vi "2FT.vi"(7 "error in":errorcluster) -> (20 "Matches (Geometric Matching 1)":T2[](array[typedef]) {"Correlation Score" format="%.2f"; "Target Template Curve Score" format="%.2f"; "Template Target Curve Score" format="%.2f"; "Bounding Box"."y" format="%.2f"; "Bounding Box"."x" format="%.2f"; "Position"."y" format="%.2f"; "Position"."x" format="%.2f"; "Score" format="%.2f"; "Scale" format="%.2f"; "Angle" format="%.2f"; "Occlusion %" format="%.2f"}, 21 "Calibrated Matches (Geometric Matching 1)":T2[](array[typedef]) {"Correlation Score" format="%.2f"; "Target Template Curve Score" format="%.2f"; "Template Target Curve Score" format="%.2f"; "Bounding Box"."y" format="%.2f"; "Bounding Box"."x" format="%.2f"; "Position"."y" format="%.2f"; "Position"."x" format="%.2f"; "Score" format="%.2f"; "Scale" format="%.2f"; "Angle" format="%.2f"; "Occlusion %" format="%.2f"}, 22 "Number of Matches (Geometric Matching 1)":i32, 27 "error out":errorcluster)   [LabVIEW 2016]
uses:
  <vilib>/vision/Pattern Matching.llb/IMAQ GM Match Report.ctl
  <vilib>/vision/Image Controls.llb/Vision Info Type2.ctl
  <vilib>/vision/Pattern Matching.llb/IMAQ Curve Parameters.ctl
  <vilib>/vision/Pattern Matching.llb/IMAQ Match Range Setting.ctl
  <vilib>/vision/driver/NI_Vision_Acquisition_Software.lvlib
  <vilib>/vision/NI_Vision_Development_Module.lvlib
panel:
  out "Image Out":T1(plugin-control)
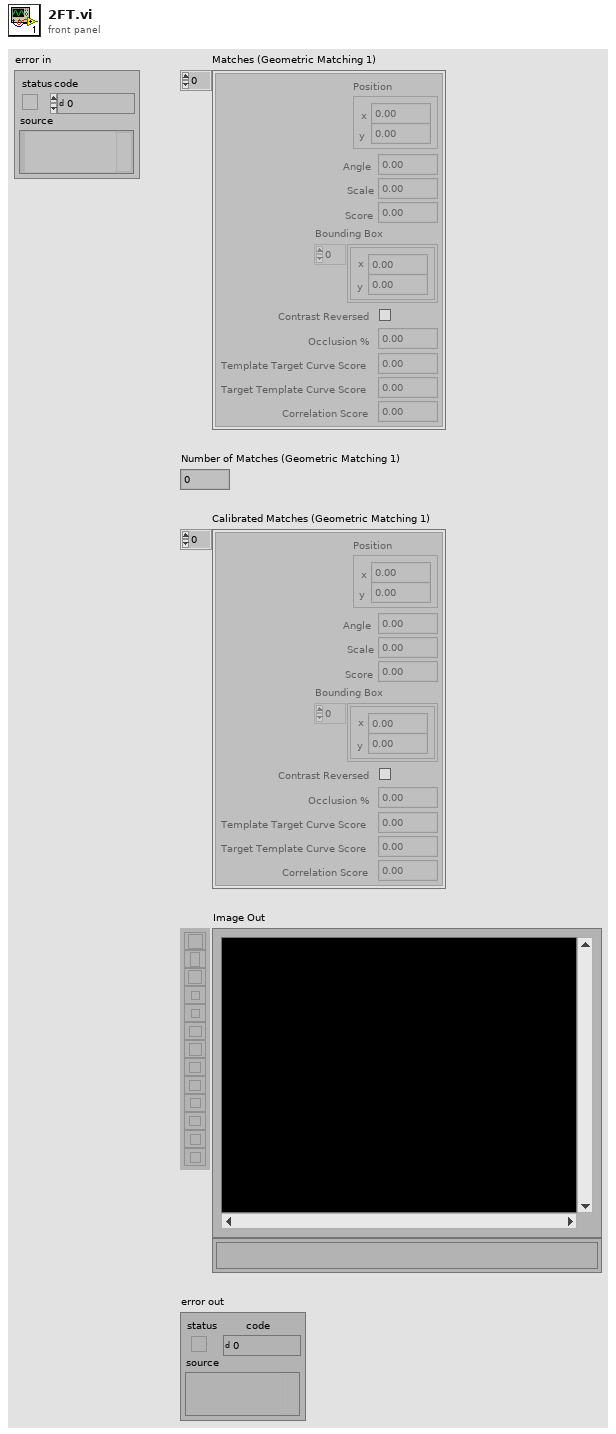
[diagram p1: front panel]
types:
  T1 = typedef "IMAQ Image.ctl" = refnum<image>
  T2 = typedef "IMAQ GM Match Report.ctl" = cluster{"Position":cluster{"x":sgl, "y":sgl}, "Angle":sgl, "Scale":sgl, "Score":sgl, "Bounding Box":cluster{"x":sgl, "y":sgl}[], "Contrast Reversed":bool, "Occlusion %":sgl, "Template Target Curve Score":sgl, "Target Template Curve Score":sgl, "Correlation Score":sgl}
  T3 = typedef "IMAQ Curve Parameters.ctl" = cluster{"Extraction Mode":u32, "Edge Threshold":i32, "Edge Filter Size":u32, "Min Length":i32, "Row Search Step Size":i32, "Col Search Step Size":i32, "Max Endpoint Gap":i32, "Closed":bool, "Subpixel":bool}
  T4 = typedef "IMAQ Match Range Setting.ctl" = cluster{"Match Constraints":u32, "Min":dbl, "Max":dbl}
  T5 = cluster{"Curve Parameters":T3, "Match Mode":cluster{"Rotation":bool, "Scale":bool, "Occlusion":bool, "Reserved":bool, "Reserved":bool, "Reserved":bool}, "Range Settings":T4[], "Number of Matches":i32, "Minimum Match Score":sgl, "SubPixel Accuracy":bool, "Adv. Geometric Match Options 2":cluster{"Setup Data Item":u16, "Item Value":dbl}[]}
  T6 = cluster{"Global Rectangle":i32[], "Contours":cluster{"ID":enum32{"External", "Internal"}, "Type":u32, "Coordinates":i32[]}[]}
  T7 = typedef "Vision Info Type2.ctl" = u32
  T8 = cluster{"Origin Pixel":cluster{"X":sgl, "Y":sgl}, "Angle Relative to Horizontal (deg)":sgl, "Axis Reference":u32}
  T9 = enum32{"AutoM", "Close", "Dilate", "Erode", "Gradient", "Gradient out", "Gradient in", "Hit miss", "Open", "PClose", "POpen", "Thick", "Thin"}
  T10 = cluster{"Brightness":sgl, "Contrast":sgl, "Gamma":sgl}
  T11 = typedef "IMAQdx.ctl" = refnum<k21>
  T12 = cluster{"histogram":u32[], "Minimal Value":sgl, "Maximal Value":sgl, "Starting Value":sgl, "Interval Width":sgl, "Mean Value":sgl, "Standard  Variation":sgl, "Area (pixels)":i32}
  T13 = typedef "Image Type" = u32
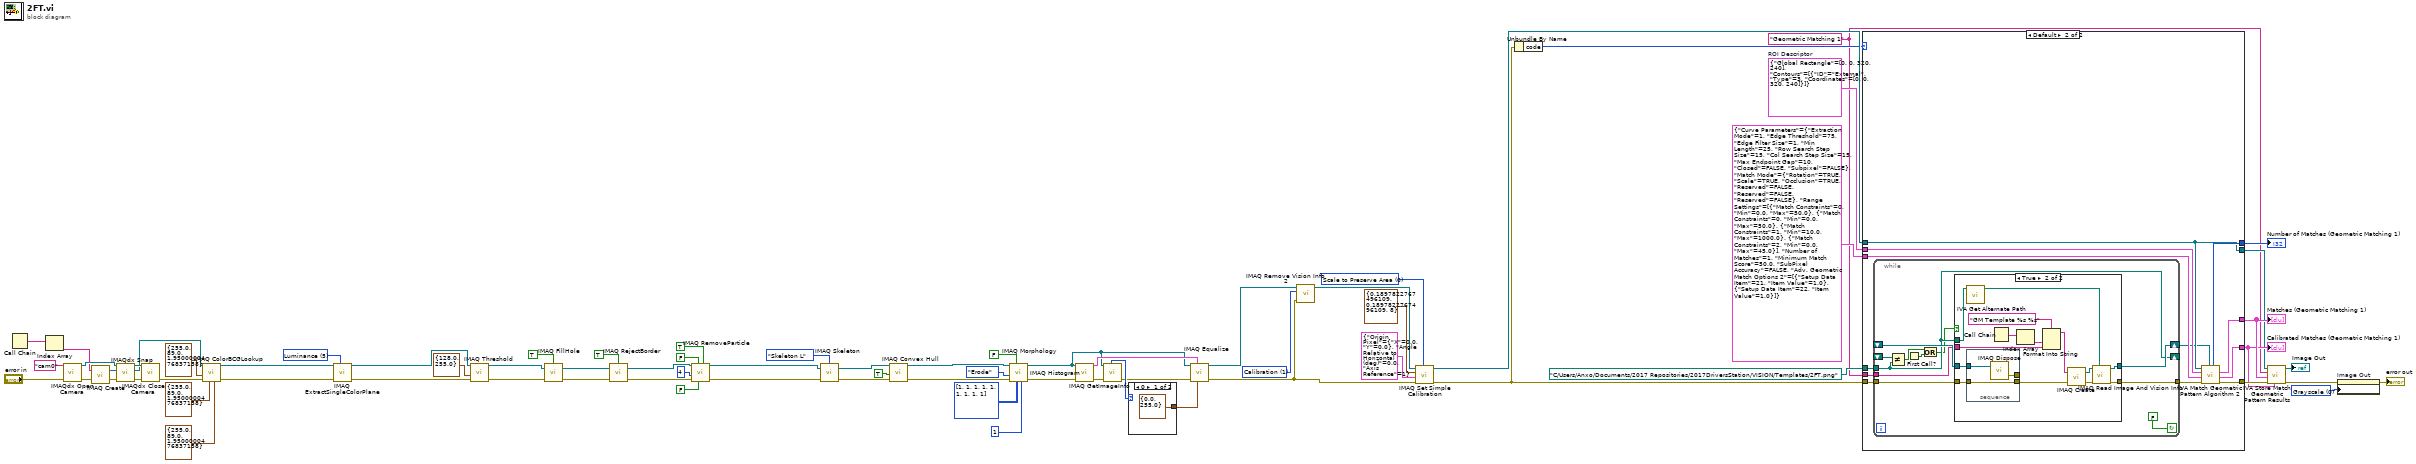
[diagram p0: block diagram]
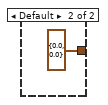
[diagram p4: hidden frame]
diagram:
  w1 = u32 0 items=["Grayscale", "Binary", "Gradient", "Rainbow", "Temperature", "User Defined", "Binary 16 Bit", "Gradient 16 Bit", "Rainbow 16 Bit", "Temperature 16 Bit", "User Defined 16 Bit"] ("Palette Type")
  w5 = "Geometric Matching 1" ("Step Name")
  w15 = T6 {"Global Rectangle"=[0, 0, 320, 240], "Contours"=[{"ID"=enum."External", "Type"=3, "Coordinates"=[0, 0, 320, 240]}]}  # ROI Descriptor
  w18 = T7 1 items=["Any", "Calibration", "Overlay", "Grayscale Template", "Color Template", "Geometric Template", "Custom Data", "Golden Template", "Geometric Template 2", "Contour Data", "Camera Model"] ("Vision Info")
  w23 = u32 0 items=["Scale to Preserve Area", "Scale to Fit"] ("Corrected Image Scaling")
  w60 = 5 items=["Red", "Green", "Blue", "Hue", "Saturation", "Luminance", "Value", "Intensity"] ("Color Plane")
  n1 = Call Chain() -> (call chain=w67:string[])
  n2 = Index Array(array=w67) -> (element=w66:string)  [unwired: 1 in]
  n3 = call <vilib>:"IMAQdx Open Camera.vi"("error in"="error in", "Session In"="cam0" ("Interface Name")) -> ("error out"=w74:errorcluster, "Session Out"=w69:T11)  [unwired: 1 in, 7 out]
  n4 = call "IMAQ Create"("Image Name"=w66, "error in (no error)"=w74) -> ("New Image"=w71:T1, "error out"=w70:errorcluster)  [unwired: 2 in, 1 out]
  n5 = call <vilib>:"IMAQdx Snap.vi"("error in"=w70, "Image In"=w71, "Session In"=w69) -> ("error out"=w72:errorcluster, "Image Out"=w65:T1, "Session Out"=w73:T11)  [unwired: 6 out]
  n6 = call <vilib>:"IMAQdx Close Camera.vi"("error in"=w72, "Session In"=w73) -> ("error out"=w64:errorcluster)  [unwired: 9 out]
  n7 = call "IMAQ ColorBCGLookup"("Blue BCG Values"=T10 {"Brightness"=255.0, "Contrast"=89.0, "Gamma"=1.95}, "Green BCG Values"=T10 {"Brightness"=255.0, "Contrast"=89.0, "Gamma"=1.95}, "error in (no error)"=w64, "Red BCG Values"=T10 {"Brightness"=255.0, "Contrast"=89.0, "Gamma"=1.95}, "Image Src"=w65) -> ("error out"=w58:errorcluster, "Image Dst Out"=w59:T1)  [unwired: 2 in, 3 out]
  n8 = call "IMAQ ExtractSingleColorPlane"("Color Plane"=w60, "error in (no error)"=w58, "Image Src"=w59) -> ("error out"=w55:errorcluster, "Image Dst Out"=w56:T1)  [unwired: 1 in, 6 out]
  n9 = call "IMAQ Threshold"("error in (no error)"=w55, "Range"=cluster{"Lower value":sgl, "Upper value":sgl} {"Lower value"=128.0, "Upper value"=255.0}, "Image Src"=w56) -> ("error out"=w52:errorcluster, "Image Dst Out"=w53:T1)  [unwired: 3 in, 4 out]
  n10 = call "IMAQ FillHole"("error in (no error)"=w52, "Image Src"=w53, "Connectivity 4/8 (8)"=TRUE) -> ("error out"=w49:errorcluster, "Image Dst Out"=w50:T1)  [unwired: 1 in, 2 out]
  n11 = call "IMAQ RejectBorder"("error in (no error)"=w49, "Image Src"=w50, "Connectivity 4/8 (8)"=TRUE) -> ("error out"=w43:errorcluster, "Image Dst Out"=w44:T1)  [unwired: 1 in, 2 out]
  n12 = call "IMAQ RemoveParticle"("Connectivity 4/8 (8)"=TRUE, "Low Pass/High Pass (Low)"=FALSE, "Square/Hexa (Square)"=FALSE, "error in (no error)"=w43, "Number of Erosion"=4, "Image Src"=w44) -> ("error out"=w40:errorcluster, "Image Dst Out"=w41:T1)  [unwired: 1 in, 3 out]
  n13 = call "IMAQ Skeleton"("error in (no error)"=w40, "Image Src"=w41, "Mode"=enum32{"Skeleton L", "Skeleton M", "Skiz"}."Skeleton L") -> ("error out"=w38:errorcluster, "Image Dst Out"=w39:T1)  [unwired: 1 in, 2 out]
  n14 = call "IMAQ Convex Hull"("error in (no error)"=w38, "Connectivity 4/8 (8)"=TRUE, "Image Src"=w39) -> ("error out"=w31:errorcluster, "Image Dst Out"=w32:T1)  [unwired: 1 in, 6 out]
  n15 = call "IMAQ Morphology"("Number of iterations (1)"=1, "Structuring Element"=i32[][] [[1, 1, 1], [1, 1, 1], [1, 1, 1]], "Square/Hexa (Square)"=FALSE, "error in (no error)"=w31, "Operation"=T9."Erode", "Image Src"=w32) -> ("error out"=w29:errorcluster, "Image Dst Out"=w27:T1)  [unwired: 1 in, 3 out]
  n16 = call "IMAQ Histogram"("error in (no error)"=w29, "Image"=w27) -> ("error out"=w26:errorcluster, "Histogram Report"=w30:T12)  [unwired: 3 in, 5 out]
  n17 = call "IMAQ GetImageInfo"("error in (no error)"=w26, "Image"=w27) -> ("error out"=w25:errorcluster, "Image Type"=w28:T13)  [unwired: 8 out]
  n18 = case shown="0" w28 {
    tunnel: [cluster{"Minimum":sgl, "Maximum":sgl} {"Minimum"=0.0, "Maximum"=255.0} ("Range") cluster{"Minimum":sgl, "Maximum":sgl} {"Minimum"=0.0, "Maximum"=0.0} ("Range")] -> w24
    frame 0 {
    }
    frame Default {
    }
  }
  n19 = call "IMAQ Equalize"("Range"=w24, "Histogram Report"=w30, "error in (no error)"=w25, "Image Src"=w27) -> ("error out"=w17:errorcluster, "Image Dst Out"=w20:T1)  [unwired: 2 in, 4 out]
  n20 = call "IMAQ Remove Vision Info 2"("error in (no error)"=w17, "Vision Info"=w18, "Image"=w20) -> ("Image Out"=w19:T1)  [unwired: 8 out]
  n21 = call "IMAQ Set Simple Calibration"("Corrected Image Scaling"=w23, "error in (no error)"=w17, "Calibration Axis Info"=T8 {"Origin Pixel"={"X"=0.0, "Y"=0.0}, "Angle Relative to Horizontal (deg)"=0.0, "Axis Reference"=1}, "Grid Descriptor"=cluster{"X Step":sgl, "Y Step":sgl, "Unit":u32} {"X Step"=0.18978228, "Y Step"=0.18978228, "Unit"=8}, "Image"=w19) -> ("error out"=w9:errorcluster, "Calibrated Image"=w14:T1)  [unwired: 1 in, 4 out]
  n22 = Unbundle By Name(w9) -> ("code"=w8:i32)
  n23 = case shown="Default" w8 {
    tunnel: path "C:/Users/Anxo/Documents/2017 Repositories/2017DriversStation/VISION/Templates/2FT.png" ("Template File Path") -> [_ w83]
    tunnel: w9 -> [_ w82]
    tunnel: T5 {"Curve Parameters"={"Extraction Mode"=1, "Edge Threshold"=75, "Edge Filter Size"=1, "Min Length"=25, "Row Search Step Size"=15, "Col Search Step Size"=15, "Max Endpoint Gap"=10, "Closed"=FALSE, "Subpixel"=FALSE}, "Match Mode"={"Rotation"=TRUE, "Scale"=TRUE, "Occlusion"=TRUE, "Reserved"=FALSE, "Reserved"=FALSE, "Reserved"=FALSE}, "Range Settings"=[{"Match Constraints"=0, "Min"=0.0, "Max"=50.0}, {"Match Constraints"=0, "Min"=0.0, "Max"=50.0}, {"Match Constraints"=1, "Min"=10.0, "Max"=1000.0}, {"Match Constraints"=2, "Min"=0.0, "Max"=45.0}], "Number of Matches"=1, "Minimum Match Score"=50.0, "SubPixel Accuracy"=FALSE, "Adv. Geometric Match Options 2"=[{"Setup Data Item"=21, "Item Value"=1.0}, {"Setup Data Item"=22, "Item Value"=1.0}]} ("Settings") -> [_ w90]
    tunnel: w15 -> [_ w89]
    tunnel: w14 -> [w78 w84]
    tunnel: [_ w88] -> w13
    tunnel: [_ w87] -> w12
    tunnel: [_ w86] -> w11
    tunnel: [_ w85] -> w10
    tunnel: [w78 w84] -> w7
    tunnel: w5 -> [_ w79]
    frame -1074396199, -1074396198 {
      # "Discard Coordinate System Error"
    }
    frame Default {
      n24 = while {
        shift-right: [w101] -> w80
        shift-left: _ -> [w100]
        tunnel: [w98] -> w81
        tunnel: w82 -> [w97]
        tunnel: w83 -> [w94]
        tunnel: w79 -> [w96]
        shift-right: [w94] -> _
        shift-left: _ -> [w95]
        stop <- FALSE continue-if-true
        n25 = Not Equal?(x=w95, y=w94) -> (x != y?=w92:bool)
        n26 = First Call?() -> (First Call?: T/F=w93:bool)
        n27 = Or(x=w92, y=w93) -> (x .or. y?=w91:bool)
        n28 = case shown="True" w91 {
          tunnel: [w103 w115] -> w101
          tunnel: w100 -> [w103 w107]
          tunnel: [w102 w112] -> w98
          tunnel: w97 -> [w102 w108]
          tunnel: w96 -> [_ w109]
          tunnel: w94 -> [_ w105]
          frame False {
          }
          frame True {
            n29 = call <vilib>:"IVA Get Alternate Path.vi"("Path In"=w105) -> ("Path Out"=w104:path)  [unwired: 10 out]
            n30 = stacked-sequence {
              tunnel: w108 -> [w120]
              tunnel: w107 -> [w119]
              tunnel: [w120] -> w106
              tunnel: [w118] -> _
              frame #0 {
                n31 = call "IMAQ Dispose"("Image"=w119) -> ("error out"=w118:errorcluster)  [unwired: 2 in, 3 out]
              }
            }
            n32 = Call Chain() -> (call chain=w111:string[])
            n33 = Index Array(array=w111) -> (element=w110:string)  [unwired: 1 in]
            n34 = Format Into String(format string="GM Template %s %s" ("Image Name"), w110, w109) -> (resulting string=w117:string)  [unwired: 2 in, 1 out]
            n35 = call "IMAQ Create"("Image Name"=w117, "error in (no error)"=w106) -> ("New Image"=w114:T1, "error out"=w113:errorcluster)  [unwired: 2 in, 1 out]
            n36 = call "IMAQ Read Image And Vision Info"("File Path"=w104, "error in (no error)"=w113, "Image"=w114) -> ("error out"=w112:errorcluster, "Image Out"=w115:T1)  [unwired: 1 in, 6 out]
          }
        }
      }
      n37 = call <vilib>:"IVA Match Geometric Pattern Algorithm 2.vi"("Template"=w80, "error in (no error)"=w81, "Settings"=w90, "ROI Descriptor"=w89, "Image"=w84) -> ("error out"=w88:errorcluster, "Calibrated Matches"=w86:T2[], "Matches"=w87:T2[], "Number of Matches"=w85:i32)  [unwired: 1 in, 2 out]
    }
  }
  "Matches (Geometric Matching 1)" <- w12
  "Number of Matches (Geometric Matching 1)" <- w10
  "Calibrated Matches (Geometric Matching 1)" <- w11
  n38 = call <vilib>:"IVA Store Match Geometric Pattern Results.vi"("Calibrated Matches"=w11, "error in (no error)"=w13, "Matches"=w12, "Step Name"=w5, "Image in"=w7) -> ("error out"=w4:errorcluster, "Image dup"=→"Image Out":T1)  [unwired: 5 out]
  n39 = property on="Image Out" class="ImageControl"(error in=w4, "Palette:Palette Type"=w1) -> (error out=→"error out":errorcluster)  [unwired: 1 in, 1 out]
